vi "Launch Consumer Relay.vi"(8 "error in (no error)":errorcluster, 9 "queueBound":i32=-1, 10 "Filter":T1={"mode"=enum."Mirror", "levelMin"=enum."INFO", "levelMax"=enum."INFO", "tagPrefix"=""}, 11 "id in":string) -> (0 "error out":errorcluster, 2 "consumerQueue":refnum<queue>, 3 "id out":string, 5 "consumerEnqueuer":refnum<class "Message Enqueuer.lvclass">)   [LabVIEW 2026, in "Tests.lvlib"]
doc: "Test-support Arrange step for message-mode relay tests. Builds a queue-mode relay appender for a given id and launches it as a standalone actor (not registered with any LogManager), returning its enqueuer and its drainable queue. Used as the consumer for a message-mode relay: the message-mode relay forwards each accepted LogStatementMsg to this enqueuer, this actor writes the Statement into its queue, and the test drains the queue to observe delivery. The consumer is test-owned: the test must stop it and destroy its queue in teardown."
uses:
  Tests.lvlib
  src/Core/Appenders/RelayAppender.lvclass/RelayAppender.lvclass
  src/TypeDefs/Severity.ctl
  src/Lumberjack.lvlib
  src/TypeDefs/DropPolicy.ctl
  src/TypeDefs/RelayMode.ctl
  <vilib>/ActorFramework/Actor/Actor.lvclass
  src/TypeDefs/FilterMode.ctl
  src/TypeDefs/Filter.ctl
  src/TypeDefs/AppenderConfig.ctl
  src/TypeDefs/Statement.ctl
  <vilib>/ActorFramework/Message Enqueuer/Message Enqueuer.lvclass
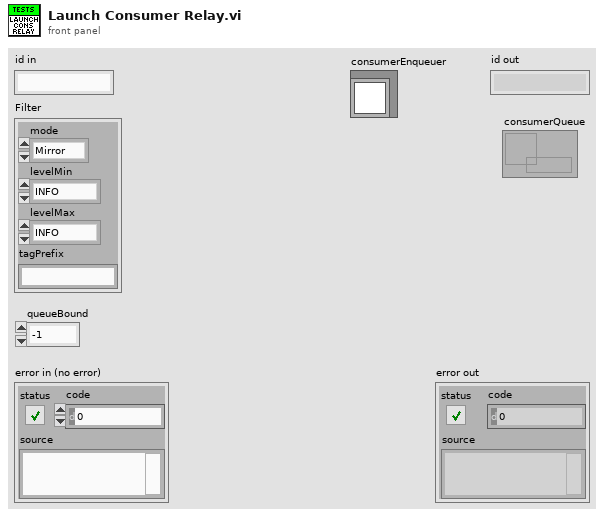
[diagram p1: front panel]
types:
  T1 = typedef "Lumberjack.lvlib/Filter.ctl" = cluster{"mode":T2, "levelMin":T3, "levelMax":T3, "tagPrefix":string}
  T2 = typedef "Lumberjack.lvlib/FilterMode.ctl" = enum16{"Mirror", "Routed"}
  T3 = typedef "Lumberjack.lvlib/Severity.ctl" = enum16{"OFF", "FATAL", "ERROR", "WARN", "INFO", "DEBUG", "TRACE", "ALL"}
  T4 = typedef "Lumberjack.lvlib/AppenderConfig.ctl" = cluster{"id":string, "threshold":T3, "filter":T1, "queueBound":i32, "dropPolicy":T5, "useUTC":bool}
  T5 = typedef "Lumberjack.lvlib/DropPolicy.ctl" = enum16{"DropOldest", "DropNewest", "LevelAware"}
  T6 = typedef "Lumberjack.lvlib/RelayMode.ctl" = enum16{"Message", "Queue"}
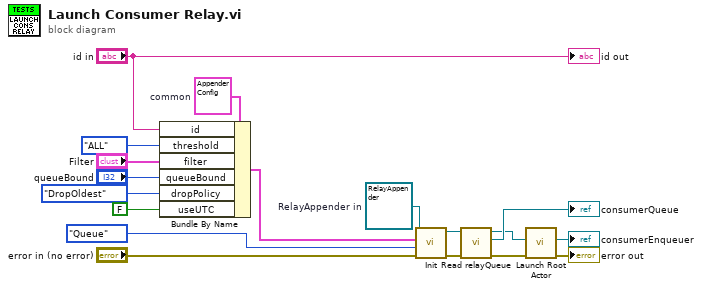
[diagram p0: block diagram]
diagram:
  w12 = T4 {"id"="", "threshold"=enum."INFO", "filter"={"mode"=enum."Mirror", "levelMin"=enum."INFO", "levelMax"=enum."INFO", "tagPrefix"=""}, "queueBound"=0, "dropPolicy"=enum."DropOldest", "useUTC"=FALSE}  # common
  w5 = refnum<class "RelayAppender.lvclass"> refnum  # RelayAppender in
  n1 = Bundle By Name(cluster=w12, "id"="id in", "threshold"=Severity."ALL" ("common.threshold"), "filter"="Filter", "queueBound"="queueBound", "dropPolicy"=DropPolicy."DropOldest" ("common.dropPolicy"), "useUTC"=FALSE ("common.useUTC")) -> (w11:T4)
  n2 = call "Init.vi"("error in (no error)"="error in (no error)", "mode"=RelayMode."Queue" ("relayMode"), "common"=w11, "RelayAppender in"=w5) -> ("error out"=w9:errorcluster, "RelayAppender out"=w8:refnum<class "RelayAppender.lvclass">)  [unwired: 6 in]
  n3 = call "Read relayQueue.vi"("error in (no error)"=w9, "RelayAppender in"=w8) -> ("error out"=w4:errorcluster, "relayQueue"=→"consumerQueue":refnum<queue>, "RelayAppender out"=w3:refnum<class "RelayAppender.lvclass">)  [unwired: 7 in]
  n4 = call <vilib>:"Launch Root Actor.vi"("error in (no error)"=w4, "Actor"=w3) -> ("error out"=→"error out":errorcluster, "Actor's Enqueuer"=→"consumerEnqueuer":refnum<class "Message Enqueuer.lvclass">)  [unwired: 8 in]
  "id out" <- "id in"
